vi "Table number type.vi"(7 "Y Scale.Display Format:Format":T1(ring), 11 "Item Names in":string[][](array[string])) -> (3 "Item Names out":string[][](array[string]))   [LabVIEW 2019, in "Report Viewer.lvlib" / "Report Viewer.lvclass"]
uses:
  Report Viewer.lvclass
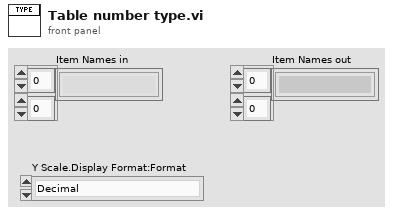
[diagram p1: front panel]
types:
  T1 = enum16{"Decimal", "Scientific", "Engineering", "Binary", "Octal", "Hexadecimal"}
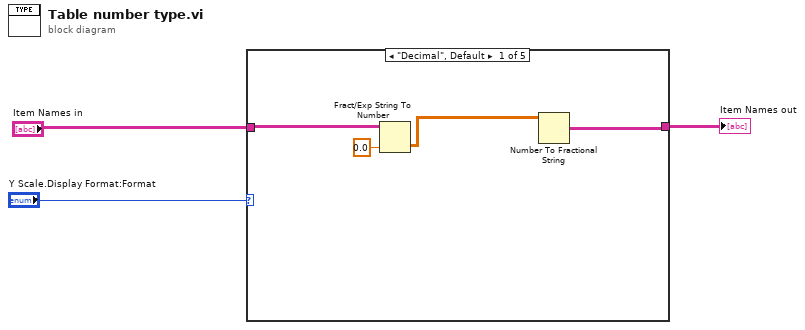
[diagram p0: block diagram]
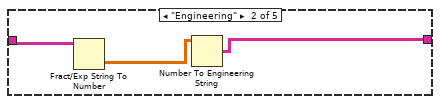
[diagram p2: hidden frame]
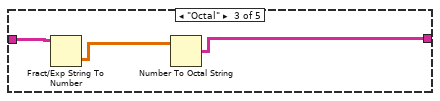
[diagram p3: hidden frame]
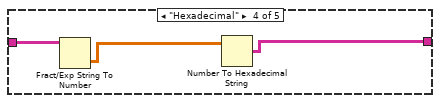
[diagram p4: hidden frame]
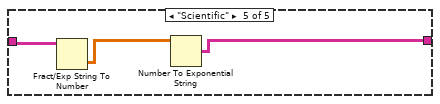
[diagram p5: hidden frame]
diagram:
  n1 = case shown="\"Decimal\", Default" "Y Scale.Display Format:Format" {
    tunnel: "Item Names in" -> [w7 w10 w13 w16 w19]
    tunnel: [w5 w8 w11 w14 w17] -> w1
    frame "Decimal", Default {
      n2 = Fract/Exp String To Number(string=w7, default (0 dbl)=0.0 ("default (0 DBL)")) -> (number=w6:dbl[][])  [unwired: 2 in, 1 out]
      n3 = Number To Fractional String(number=w6) -> (F-format string=w5:string[][])  [unwired: 3 in]
    }
    frame "Engineering" {
      n4 = Fract/Exp String To Number(string=w10) -> (number=w9:dbl[][])  [unwired: 3 in, 1 out]
      n5 = Number To Engineering String(4:w9) -> (0:w8:string[][])  [unwired: 3 in]
    }
    frame "Octal" {
      n6 = Fract/Exp String To Number(string=w13) -> (number=w12:dbl[][])  [unwired: 3 in, 1 out]
      n7 = Number To Octal String(2:w12) -> (0:w11:string[][])  [unwired: 1 in]
    }
    frame "Hexadecimal" {
      n8 = Fract/Exp String To Number(string=w16) -> (number=w15:dbl[][])  [unwired: 3 in, 1 out]
      n9 = Number To Hexadecimal String(2:w15) -> (0:w14:string[][])  [unwired: 1 in]
    }
    frame "Scientific" {
      n10 = Fract/Exp String To Number(string=w19) -> (number=w18:dbl[][])  [unwired: 3 in, 1 out]
      n11 = Number To Exponential String(number=w18) -> (E-format string=w17:string[][])  [unwired: 3 in]
    }
  }
  "Item Names out" <- w1
